vi "HEWH Check Test Complete.vi"(0 "Test Patten Setup.PRAT/RLT Sequence":T1[](array[typedef]) {"Time" format="%<%H:%M:%S>t"}, 5 "A Timer":dbl, 11 "Error In":errorcluster, 12 "Current Sequence":T1={"Sequence #"=0.0, "Cycles"=0, "Mode Setting"="", "Flow Rate (GPM)"=0.0, "Temperature (F)"=0.0, "Reset Timer"=FALSE, "Use Temp Decline Method"=FALSE, "Terminate Condition"=enum."C1-Terminate Draw @ Gallon Mark", "Condition Value #1"=0.0, "UE"=FALSE, "LE"=FALSE, "Comp"=FALSE, "Fan"=FALSE, "Test End Time (Sec)"=0.0, "Purge Until Cutout"=FALSE, "Start Conditions"=enum."Heat Source Cutout", "Condition Value #2"=0.0, "Remove Power"=FALSE, "Time"=0.0, "Check Special Cond."=enum."SC2-Check Heat Source (On-C2/Off-C1)", "Condition#"=enum."C1", "Draw Flags"=enum."N/A", "Data Processing Delay (FHD 15sec, UEF 5 Sec)"=0.0, "Test Complete"=FALSE} {"Time" format="%<%H:%M:%S>t"}) -> (1 "Do NOT Check Timer":bool, 3 "Test Complete":bool, 4 "Last Draw Condition Output":T1={"Sequence #"=0.0, "Cycles"=0, "Mode Setting"="", "Flow Rate (GPM)"=0.0, "Temperature (F)"=0.0, "Reset Timer"=FALSE, "Use Temp Decline Method"=FALSE, "Terminate Condition"=enum."C1-Terminate Draw @ Gallon Mark", "Condition Value #1"=0.0, "UE"=FALSE, "LE"=FALSE, "Comp"=FALSE, "Fan"=FALSE, "Test End Time (Sec)"=0.0, "Purge Until Cutout"=FALSE, "Start Conditions"=enum."Heat Source Cutout", "Condition Value #2"=0.0, "Remove Power"=FALSE, "Time"=0.0, "Check Special Cond."=enum."SC2-Check Heat Source (On-C2/Off-C1)", "Condition#"=enum."C1", "Draw Flags"=enum."N/A", "Data Processing Delay (FHD 15sec, UEF 5 Sec)"=0.0, "Test Complete"=FALSE} {"Time" format="%<%H:%M:%S>t"}, 6 "Seconds Remaining":dbl, 8 "Disable Station":bool, 10 "Use Last Start Condition?":bool, 14 "Start Conditions":T4, 15 "Error Out":errorcluster)   [LabVIEW 2016]
uses:
  Type Definitions/HEWH Start Conditions.ctl
  Type Definitions/PRAT Test.ctl
  Utility/Save File/File Setup (Public)/Type Definition/Save File HEWH Heating Control Mode.ctl
  Draw Water Specific/Type Definitions/Terminate Draw Conditions.ctl
  Draw Water Specific/Type Definitions/Check Special Condtions.ctl
  Draw Water Specific/Type Definitions/HEWH Special Condition Check.ctl
  Type Definitions/HEWH Draw Flag ENUM.ctl
  Utility/Type Definitions/UTILITY Notifier.ctl
  Utility/Save File/File Setup.lvlib
panel:
  in  "Debug":T1[](array[typedef])=[{"Sequence #"=1.0, "Cycles"=1, "Mode Setting"="", "Flow Rate (GPM)"=3.0, "Temperature (F)"=58.0, "Reset Timer"=FALSE, "Use Temp Decline Method"=FALSE, "Terminate Condition"=enum."C7-Until Any Heat Source", "Condition Value #1"=0.0, "UE"=FALSE, "LE"=FALSE, "Comp"=FALSE, "Fan"=FALSE, "Test End Time (Sec)"=0.0, "Purge Until Cutout"=FALSE, "Start Conditions"=enum."Heat Source Cutout", "Condition Value #2"=0.0, "Remove Power"=FALSE, "Time"=0.0, "Check Special Cond."=enum."SC2-Check Heat Source (On-C2/Off-C1)", "Condition#"=enum."C1", "Draw Flags"=enum."N/A", "Data Processing Delay (FHD 15sec, UEF 5 Sec)"=0.0, "Test Complete"=FALSE}, {"Sequence #"=2.0, "Cycles"=1, "Mode Setting"="", "Flow Rate (GPM)"=3.0, "Temperature (F)"=58.0, "Reset Timer"=TRUE, "Use Temp Decline Method"=TRUE, "Terminate Condition"=enum."C1-Terminate Draw @ Gallon Mark", "Condition Value #1"=0.0, "UE"=FALSE, "LE"=FALSE, "Comp"=FALSE, "Fan"=FALSE, "Test End Time (Sec)"=0.0, "Purge Until Cutout"=FALSE, "Start Conditions"=enum."At Time (Seconds)", "Condition Value #2"=0.0, "Remove Power"=FALSE, "Time"=0.0, "Check Special Cond."=enum."SC2-Check Heat Source (On-C2/Off-C1)", "Condition#"=enum."C1", "Draw Flags"=enum."N/A", "Data Processing Delay (FHD 15sec, UEF 5 Sec)"=0.0, "Test Complete"=FALSE}, {"Sequence #"=3.0, "Cycles"=1, "Mode Setting"="", "Flow Rate (GPM)"=3.0, "Temperature (F)"=58.0, "Reset Timer"=FALSE, "Use Temp Decline Method"=FALSE, "Terminate Condition"=enum."C1-Terminate Draw @ Gallon Mark", "Condition Value #1"=0.0, "UE"=FALSE, "LE"=FALSE, "Comp"=FALSE, "Fan"=FALSE, "Test End Time (Sec)"=0.0, "Purge Until Cutout"=FALSE, "Start Conditions"=enum."At Time (Seconds)", "Condition Value #2"=0.0, "Remove Power"=FALSE, "Time"=0.0, "Check Special Cond."=enum."SC2-Check Heat Source (On-C2/Off-C1)", "Condition#"=enum."C1", "Draw Flags"=enum."N/A", "Data Processing Delay (FHD 15sec, UEF 5 Sec)"=0.0, "Test Complete"=FALSE}, {"Sequence #"=4.0, "Cycles"=1, "Mode Setting"="", "Flow Rate (GPM)"=3.0, "Temperature (F)"=58.0, "Reset Timer"=FALSE, "Use Temp Decline Method"=FALSE, "Terminate Condition"=enum."C1-Terminate Draw @ Gallon Mark", "Condition Value #1"=0.0, "UE"=FALSE, "LE"=FALSE, "Comp"=FALSE, "Fan"=FALSE, "Test End Time (Sec)"=0.0, "Purge Until Cutout"=FALSE, "Start Conditions"=enum."At Time (Seconds)", "Condition Value #2"=0.0, "Remove Power"=FALSE, "Time"=0.0, "Check Special Cond."=enum."SC2-Check Heat Source (On-C2/Off-C1)", "Condition#"=enum."C1", "Draw Flags"=enum."N/A", "Data Processing Delay (FHD 15sec, UEF 5 Sec)"=0.0, "Test Complete"=FALSE}, {"Sequence #"=5.0, "Cycles"=1, "Mode Setting"="", "Flow Rate (GPM)"=3.0, "Temperature (F)"=58.0, "Reset Timer"=FALSE, "Use Temp Decline Method"=FALSE, "Terminate Condition"=enum."C1-Terminate Draw @ Gallon Mark", "Condition Value #1"=0.0, "UE"=FALSE, "LE"=FALSE, "Comp"=FALSE, "Fan"=FALSE, "Test End Time (Sec)"=0.0, "Purge Until Cutout"=FALSE, "Start Conditions"=enum."At Time (Seconds)", "Condition Value #2"=0.0, "Remove Power"=FALSE, "Time"=0.0, "Check Special Cond."=enum."SC2-Check Heat Source (On-C2/Off-C1)", "Condition#"=enum."C1", "Draw Flags"=enum."N/A", "Data Processing Delay (FHD 15sec, UEF 5 Sec)"=0.0, "Test Complete"=FALSE}, {"Sequence #"=6.0, "Cycles"=1, "Mode Setting"="", "Flow Rate (GPM)"=3.0, "Temperature (F)"=58.0, "Reset Timer"=FALSE, "Use Temp Decline Method"=FALSE, "Terminate Condition"=enum."C1-Terminate Draw @ Gallon Mark", "Condition Value #1"=0.0, "UE"=FALSE, "LE"=FALSE, "Comp"=FALSE, "Fan"=FALSE, "Test End Time (Sec)"=0.0, "Purge Until Cutout"=FALSE, "Start Conditions"=enum."At Time (Seconds)", "Condition Value #2"=0.0, "Remove Power"=FALSE, "Time"=0.0, "Check Special Cond."=enum."SC2-Check Heat Source (On-C2/Off-C1)", "Condition#"=enum."C1", "Draw Flags"=enum."N/A", "Data Processing Delay (FHD 15sec, UEF 5 Sec)"=0.0, "Test Complete"=FALSE}, {"Sequence #"=7.0, "Cycles"=1, "Mode Setting"="", "Flow Rate (GPM)"=3.0, "Temperature (F)"=58.0, "Reset Timer"=FALSE, "Use Temp Decline Method"=FALSE, "Terminate Condition"=enum."C1-Terminate Draw @ Gallon Mark", "Condition Value #1"=0.0, "UE"=FALSE, "LE"=FALSE, "Comp"=FALSE, "Fan"=FALSE, "Test End Time (Sec)"=86400.0, "Purge Until Cutout"=FALSE, "Start Conditions"=enum."At Time (Seconds)", "Condition Value #2"=0.0, "Remove Power"=FALSE, "Time"=0.0, "Check Special Cond."=enum."SC2-Check Heat Source (On-C2/Off-C1)", "Condition#"=enum."C1", "Draw Flags"=enum."N/A", "Data Processing Delay (FHD 15sec, UEF 5 Sec)"=0.0, "Test Complete"=FALSE}] {"Time" format="%<%H:%M:%S>t"}
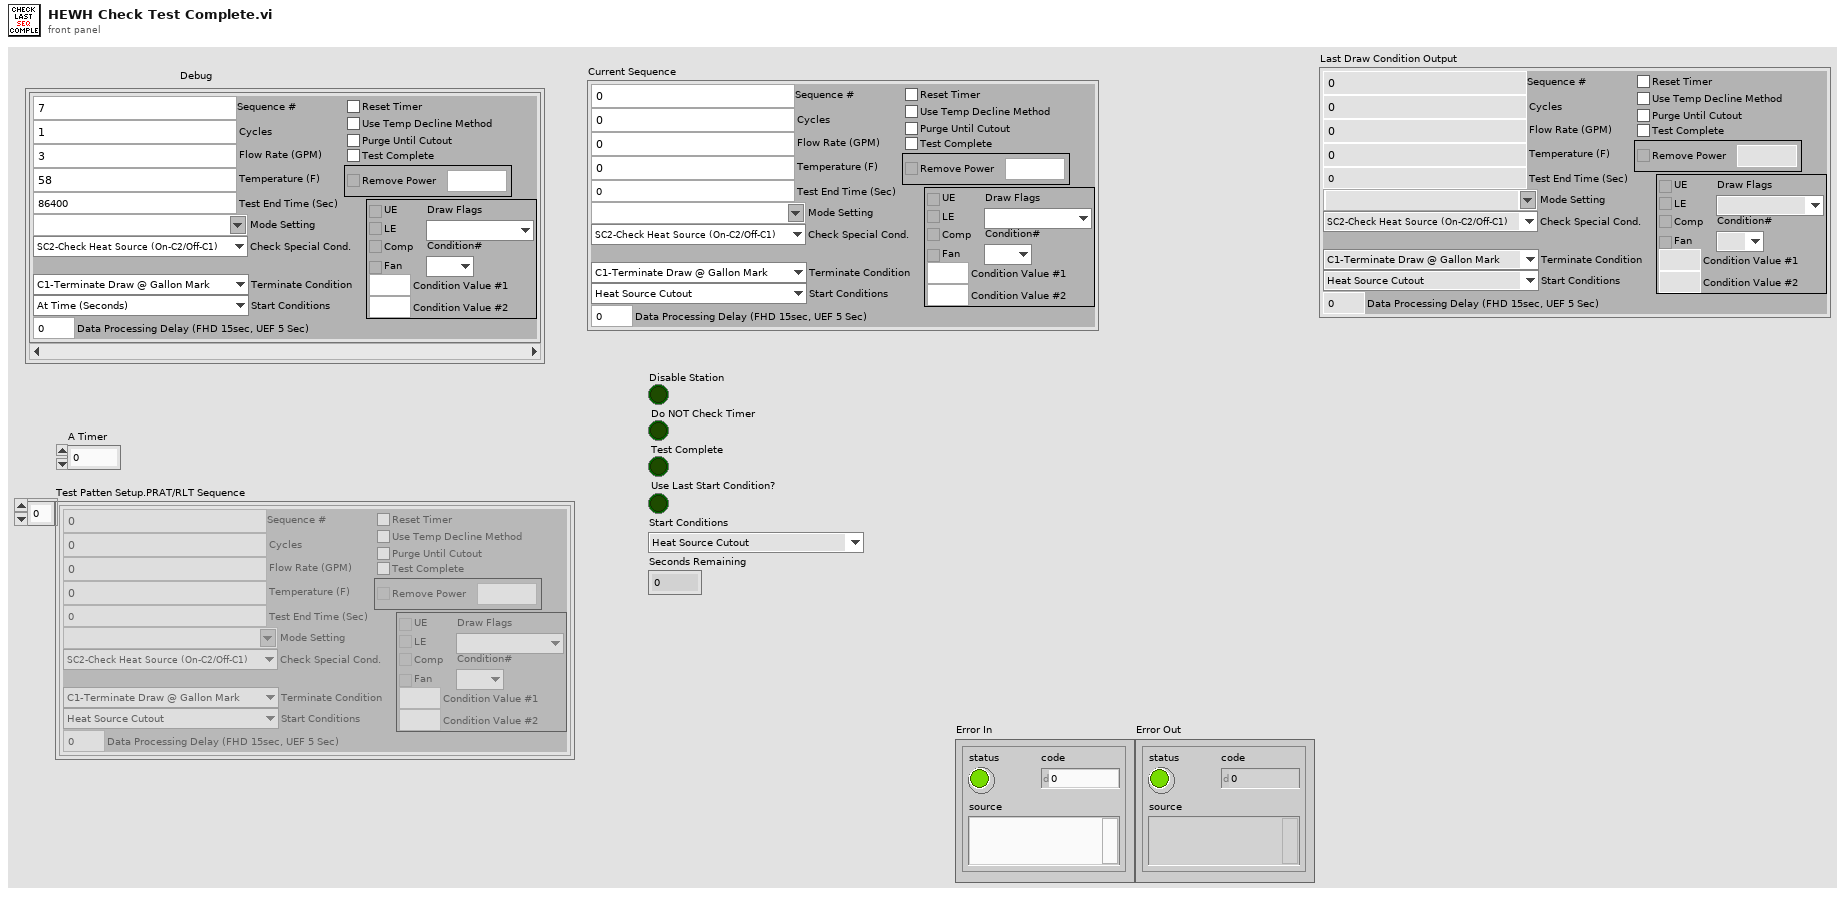
[diagram p1: front panel]
types:
  T1 = typedef "PRAT Test.ctl" = cluster{"Sequence #":dbl, "Cycles":i32, "Mode Setting":T2, "Flow Rate (GPM)":dbl, "Temperature (F)":dbl, "Reset Timer":bool, "Use Temp Decline Method":bool, "Terminate Condition":T3, "Condition Value #1":dbl, "UE":bool, "LE":bool, "Comp":bool, "Fan":bool, "Test End Time (Sec)":dbl, "Purge Until Cutout":bool, "Start Conditions":T4, "Condition Value #2":dbl, "Remove Power":bool, "Time":dbl, "Check Special Cond.":T5, "Condition#":T6, "Draw Flags":T7, "Data Processing Delay (FHD 15sec, UEF 5 Sec)":dbl, "Test Complete":bool}
  T2 = typedef "File Setup.lvlib/Save File HEWH Heating Control Mode.ctl" = string
  T3 = typedef "Terminate Draw Conditions.ctl" = enum16{"C1-Terminate Draw @ Gallon Mark", "C2-Special Last Draw (HU Test)", "C3-RTD Out <=", "C4-Mean Tank Temp <=", "C5-Decrease RTD Out (Deg F)", "C6-Time (Seconds)", "C7-Until Any Heat Source", "C8-Specific Heat Source", "C9-Do Nothing"}
  T4 = typedef "HEWH Start Conditions.ctl" = enum16{"Heat Source Cutout", "At Time (Seconds)", "Every X (Seconds)", "T2 >= X° Below Setpoint", "Seconds From Complete", "Wait for LE & Comp Cutout", "Wait for Comp Cutout", "Wait for LE Cutout", "Wait for UE Cutout"}
  T5 = typedef "Check Special Condtions.ctl" = enum16{"SC1-Do Nothing", "SC2-Check Heat Source (On-C2/Off-C1)", "SC3-Check Skip Condition", "SC4-Check Heat Source ON/Fail"}
  T6 = typedef "HEWH Special Condition Check.ctl" = enum16{"N/A", "C1", "C2", "Reset/Fail", "Skip Draw Sequence"}
  T7 = typedef "HEWH Draw Flag ENUM.ctl" = enum16{"N/A", "None(0)", "Sml(1)", "Med(2)", "SmlMed(3)", "Lrg(4)", "SmlLrg(5)", "MedLrg(6)", "SmlMedLrg(7)"}
  T8 = typedef "UTILITY Notifier.ctl" = enum16{"Set", "Read", "Release Ref"}
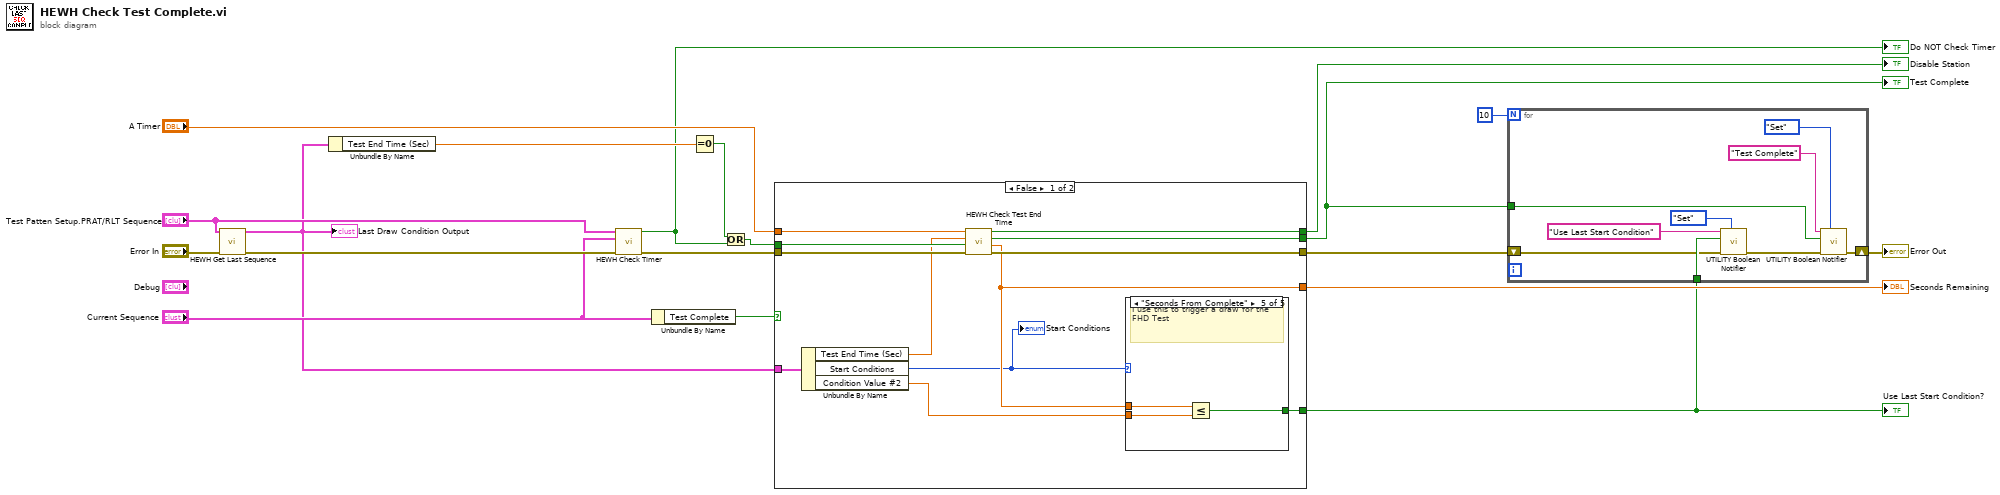
[diagram p0: block diagram]
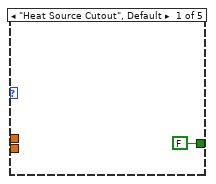
[diagram p2: hidden frame]
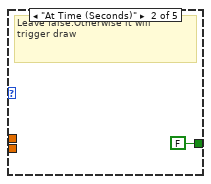
[diagram p3: hidden frame]
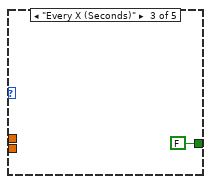
[diagram p4: hidden frame]
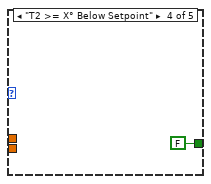
[diagram p5: hidden frame]
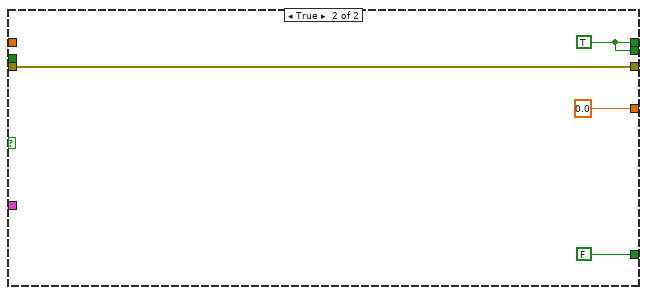
[diagram p6: hidden frame]
diagram:
  n1 = call "HEWH Get Last Sequence.vi"("Error In"="Error In", "Test Patten Setup.PRAT/RLT Sequence"="Test Patten Setup.PRAT/RLT Sequence") -> ("Error Out"=w13:errorcluster, "Last Sequence"=w2:T1)  [unwired: 7 in, 1 out]
  "Last Draw Condition Output" <- w2
  n2 = Unbundle By Name(w2) -> ("Test End Time (Sec)"=w18:dbl)
  n3 = call "HEWH Check Timer.vi"("Error In"=w13, "Current Sequence"="Current Sequence", "Test Patten Setup.PRAT/RLT Sequence"="Test Patten Setup.PRAT/RLT Sequence") -> ("Error Out"=w8:errorcluster, "Do NOT Check Timer"=w14:bool)  [unwired: 7 in]
  "Do NOT Check Timer" <- w14
  n4 = Unbundle By Name("Current Sequence") -> ("Test Complete"=w3:bool)
  n5 = Equal To 0?(x=w18) -> (x = 0?=w16:bool)
  n6 = Or(x=w16, y=w14) -> (x .or. y?=w15:bool)
  n7 = case shown="False" w3 {
    tunnel: "A Timer" -> [w31 _]
    tunnel: w15 -> [w30 _]
    tunnel: [w29 w42] -> w11
    tunnel: [w28 w42] -> w9
    tunnel: w8 -> [w27 w41]
    tunnel: [w26 w41] -> w7
    tunnel: [w22 0.0 ("Seconds Remaining")] -> w5
    tunnel: w2 -> [w25 _]
    tunnel: [w20 FALSE] -> w1
    frame False {
      n8 = Unbundle By Name(w25) -> ("Test End Time (Sec)"=w23:dbl, "Start Conditions"=w21:T4, "Condition Value #2"=w24:dbl)
      "Start Conditions" <- w21
      n9 = call "HEWH Check Test End Time.vi"("Error In"=w27, "Do NOT Check Timer"=w30, "Test End Time (Sec)"=w23, "A Timer"=w31) -> ("Error Out"=w26:errorcluster, "Seconds Remaining"=w22:dbl, "Test Complete"=w29:bool, "Disable Station"=w28:bool)  [unwired: 4 in]
      n10 = case shown="\"Seconds From Complete\"" w21 {
        tunnel: w24 -> [_ _ _ _ w37]
        tunnel: w22 -> [_ _ _ _ w38]
        tunnel: [FALSE FALSE FALSE FALSE w36] -> w20
        frame "Heat Source Cutout", Default {
        }
        frame "At Time (Seconds)" {
          # "Leave false.Otherwise it will\ntrigger draw"
        }
        frame "Every X (Seconds)" {
        }
        frame "T2 >= X° Below Setpoint" {
        }
        frame "Seconds From Complete" {
          # "I use this to trigger a draw for the FHD Test"
          n11 = Less Or Equal?(x=w38, y=w37) -> (x <= y?=w36:bool)
        }
      }
    }
    frame True {
      w42 = TRUE ("Disable Station")
    }
  }
  "Use Last Start Condition?" <- w1
  "Seconds Remaining" <- w5
  "Test Complete" <- w11
  "Disable Station" <- w9
  n12 = for {
    N: 10 -> [_]
    tunnel: w1 -> [w49]
    tunnel: w11 -> [w43]
    shift-right: [w44] -> w12
    shift-left: w7 -> [w48]
    n13 = call "UTILITY Boolean Notifier.vi"("Status"=UTILITY_Notifier."Set", "error in (no error)"=w48, "Set Status"=w49, "name (unnamed)"="Use Last Start Condition") -> ("error out"=w45:errorcluster)  [unwired: 6 in, 1 out]
    n14 = call "UTILITY Boolean Notifier.vi"("Status"=UTILITY_Notifier."Set", "error in (no error)"=w45, "Set Status"=w43, "name (unnamed)"="Test Complete") -> ("error out"=w44:errorcluster)  [unwired: 6 in, 1 out]
  }
  "Error Out" <- w12
